vi "loadSettings.vi"(8 "error in (no error)":errorcluster, 10 "Path":path, 11 "WinX32Settings in":refnum<class "WinX32Settings.lvclass">) -> (0 "error out":errorcluster, 3 "WinX32Settings out":refnum<class "WinX32Settings.lvclass">)   [LabVIEW 2011, in "Tools.lvlib" / "Settings.lvlib" / "WinX32Settings.lvclass"]
uses:
  WinX32Settings.lvclass
  WinX32Settings.lvclass/WinX32Settings.ctl
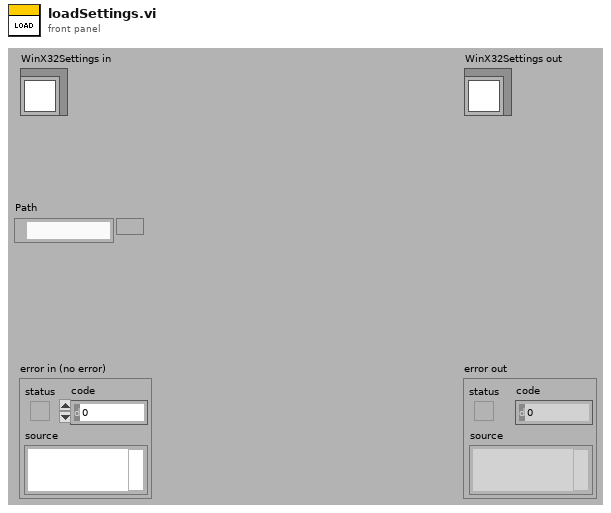
[diagram p1: front panel]
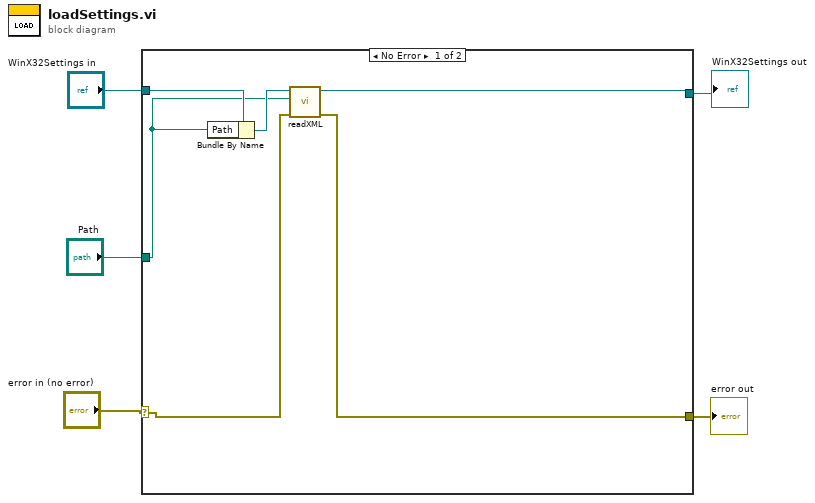
[diagram p0: block diagram]
diagram:
  n1 = case shown="No Error" "error in (no error)" {
    selector: "error in (no error)" -> [w9 w13]
    tunnel: [w7 w13] -> w4
    tunnel: [w8 w12] -> w2
    tunnel: "WinX32Settings in" -> [w11 w12]
    tunnel: "Path" -> [w6 _]
    frame No Error {
      n2 = Bundle By Name(cluster=w11, "Path"=w6) -> (w10:refnum<class "WinX32Settings.lvclass">)
      n3 = call "readXML.vi"("error in (no error)"=w9, "Path"=w6, "WinX32Settings in"=w10) -> ("error out"=w7:errorcluster, "WinX32Settings out"=w8:refnum<class "WinX32Settings.lvclass">)  [unwired: 7 in]
    }
    frame Error {
    }
  }
  "error out" <- w4
  "WinX32Settings out" <- w2
